vi "DHE_SetControllerStatus.vi"(9 "framesperbuffer":i32, 10 "ControllerStatus":T1={"Response"="", "power"=FALSE, "shutter"=FALSE, "artifdata"=FALSE, "idlemode"=FALSE, "reset"=FALSE, "gain"=0, "speed"=0, "resetPCI"=FALSE, "autoshutter"=FALSE, "TempSetPoint"=-110, "multipleextensions"=FALSE, "displayImage"=TRUE, "coadding"=FALSE, "images being coadded"=1, "Operation Mode"=enum."normal", "frames to write"={"subs"=FALSE, "reset"=FALSE, "exposed"=FALSE}, "fawler samples"=1, "write auto"=FALSE, "datatype"="", "frames to display"={"subs"=FALSE, "reset"=FALSE, "exposed"=FALSE}, "sur"=1, "autoclear"=FALSE}) -> ()   [LabVIEW 2016]
uses:
  Common/public/vis/CMN_ContStatus.ctl
  DBSHAND/private/vis/DatabaseHand_Element_Set(bool).vi
  DBSHAND/private/vis/DatabaseHand_Element_Set(U8).vi
  DBSHAND/private/vis/DatabaseHand_Element_Set(I32).vi
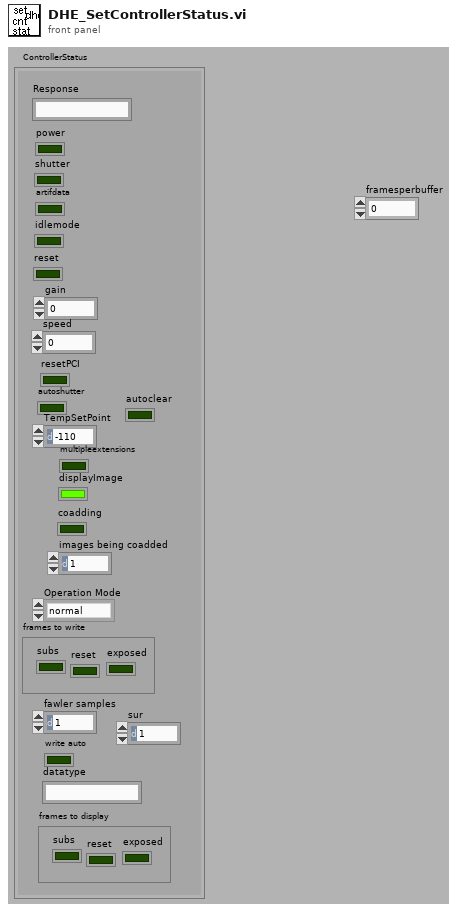
[diagram p1: front panel]
types:
  T1 = typedef "CMN_ContStatus.ctl" = cluster{"Response":string, "power":bool, "shutter":bool, "artifdata":bool, "idlemode":bool, "reset":bool, "gain":u8, "speed":u8, "resetPCI":bool, "autoshutter":bool, "TempSetPoint":i32, "multipleextensions":bool, "displayImage":bool, "coadding":bool, "images being coadded":i32, "Operation Mode":enum16{"normal", "coadd", "fawler"}, "frames to write":cluster{"subs":bool, "reset":bool, "exposed":bool}, "fawler samples":i32, "write auto":bool, "datatype":string, "frames to display":cluster{"subs":bool, "reset":bool, "exposed":bool}, "sur":i32, "autoclear":bool}
  T2 = typedef "DatabaseHand_RefNum.ctl" = refnum<vi>
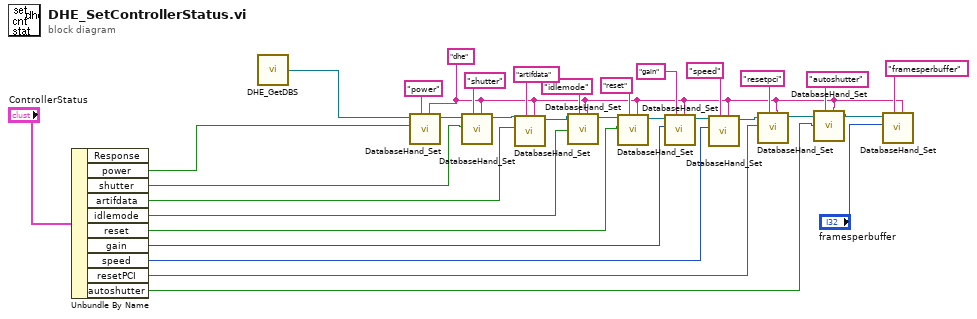
[diagram p0: block diagram]
diagram:
  w2 = "dhe" ("group")
  n1 = Unbundle By Name("ControllerStatus") -> ("power"=w30:bool, "shutter"=w24:bool, "artifdata"=w22:bool, "idlemode"=w20:bool, "reset"=w18:bool, "gain"=w7:u8, "speed"=w6:u8, "resetPCI"=w17:bool, "autoshutter"=w15:bool)  [unwired: 1 out]
  n2 = call "DHE_GetDBS.vi"() -> ("DHE_DBSRef"=w1:T2)  [unwired: 9 out]
  n3 = call-poly "DatabaseHand_Set.vi"("group"=w2, "name"="power", "value"=w30, "Database RefNum in"=w1) -> ("Database RefNum out"=w29:T2)  [unwired: 4 in, 3 out]
  n4 = call-poly "DatabaseHand_Set.vi"("group"=w2, "name"="shutter", "value"=w24, "Database RefNum in"=w29) -> ("Database RefNum out"=w28:T2)  [unwired: 4 in, 3 out]
  n5 = call-poly "DatabaseHand_Set.vi"("group"=w2, "name"="artifdata", "value"=w22, "Database RefNum in"=w28) -> ("Database RefNum out"=w27:T2)  [unwired: 4 in, 3 out]
  n6 = call-poly "DatabaseHand_Set.vi"("group"=w2, "name"="idlemode", "value"=w20, "Database RefNum in"=w27) -> ("Database RefNum out"=w26:T2)  [unwired: 4 in, 3 out]
  n7 = call-poly "DatabaseHand_Set.vi"("group"=w2, "name"="reset", "value"=w18, "Database RefNum in"=w26) -> ("Database RefNum out"=w12:T2)  [unwired: 4 in, 3 out]
  n8 = call-poly "DatabaseHand_Set.vi"("group"=w2, "name"="gain", "value"=w7, "Database RefNum in"=w12) -> ("Database RefNum out"=w11:T2)  [unwired: 4 in, 3 out]
  n9 = call-poly "DatabaseHand_Set.vi"("group"=w2, "name"="speed", "value"=w6, "Database RefNum in"=w11) -> ("Database RefNum out"=w10:T2)  [unwired: 4 in, 3 out]
  n10 = call-poly "DatabaseHand_Set.vi"("group"=w2, "name"="resetpci", "value"=w17, "Database RefNum in"=w10) -> ("Database RefNum out"=w25:T2)  [unwired: 4 in, 3 out]
  n11 = call-poly "DatabaseHand_Set.vi"("group"=w2, "name"="autoshutter", "value"=w15, "Database RefNum in"=w25) -> ("Database RefNum out"=w5:T2)  [unwired: 4 in, 3 out]
  n12 = call-poly "DatabaseHand_Set.vi"("group"=w2, "name"="framesperbuffer", "value"="framesperbuffer", "Database RefNum in"=w5) -> ()  [unwired: 4 in, 4 out]
